vi "Sub_IR_front_rechts.vi"(10 "Geschwindigkeit manuel":dbl(knob) scale=0.0..1.0, 11 "Neue/alte Formel":bool) -> (3 "Geschw_IR_vorne":dbl)   [LabVIEW 2016]
doc: "Geschwindigkeitsregelung anhand IR Sensor vorne\n05.04.17_Tloe"
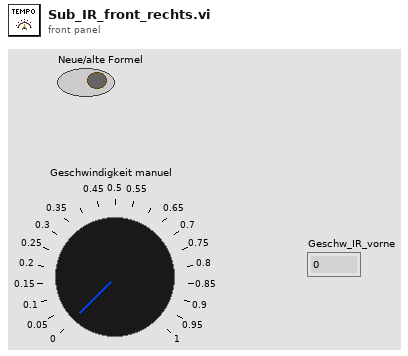
[diagram p1: front panel]
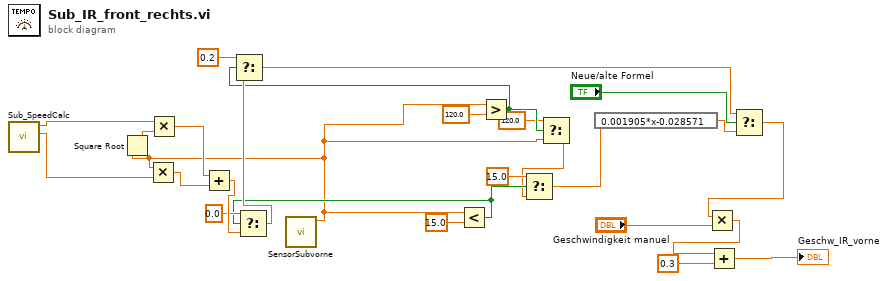
[diagram p0: block diagram]
diagram:
  n1 = call "Sub_SpeedCalc.vi"() -> ("a"=w13:dbl, "b"=w14:dbl)  [unwired: 8 in]
  n2 = call "SensorSubvorne.vi"() -> ("Abstand in cm"=w11:dbl)  [unwired: 9 in, 2 out]
  n3 = Square Root(x=w11) -> (sqrt(x)=w12:dbl)
  n4 = Multiply(x=w11, y=w14) -> (x*y=w16:dbl)
  n5 = Multiply(x=w13, y=w12) -> (x*y=w15:dbl)
  n6 = Add(x=w15, y=w16) -> (x+y=w21:dbl)
  n7 = Less?(x=w11, y=15.0) -> (x < y?=w19:bool)
  n8 = Select(t=0.0, s=w19, f=w21) -> (s? t:f=w22:dbl)
  n9 = Greater?(x=w11, y=120.0) -> (0:w17:bool)
  n10 = Select(t=0.2, s=w17, f=w22) -> (s? t:f=w25:dbl)
  n11 = Select(t=120.0, s=w17, f=w11) -> (s? t:f=w5:dbl)
  n12 = Select(t=15.0, s=w19, f=w5) -> (s? t:f=w8:dbl)
  n13 = expression code="0.001905*x-0.028571"(w8) -> (w24:dbl)
  n14 = Select(t=w25, s="Neue/alte Formel", f=w24) -> (s? t:f=w23:dbl)
  n15 = Multiply(x=w23, y="Geschwindigkeit manuel") -> (x*y=w9:dbl)
  n16 = Add(x=w9, y=0.3) -> (x+y=→"Geschw_IR_vorne":dbl)
